vi "Flatten modbus object to byte array.vi"(11 "Object":T1 {"Object ID" format="%x"}) -> (3 "byte array":u8[](array[numeric]))   [LabVIEW 2021, in "Device Data Model.lvclass"]
uses:
  Device Data Model.lvclass
  Identification Parameters.ctl
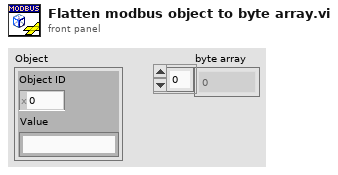
[diagram p1: front panel]
types:
  T1 = typedef "Device Data Model.lvclass/Identification Parameters.ctl" = cluster{"Object ID":u8, "Value":string}
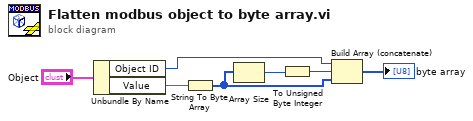
[diagram p0: block diagram]
diagram:
  n1 = Unbundle By Name("Object") -> ("Object ID"=w5:u8, "Value"=w2:string)
  n2 = String To Byte Array(string=w2) -> (unsigned byte array=w4:u8[])
  n3 = Array Size(array=w4) -> (size(s)=w3:i32)
  n4 = To Unsigned Byte Integer(number=w3) -> (unsigned 8bit integer=w6:u8)
  n5 = Build Array (concatenate)(w5, w6, w4) -> (→"byte array":u8[])
